vi "Lab Panel V4.86.vi"() -> ()   [LabVIEW 2013] (continued)
                            n1529 = local write "DISP LAB03-2"(w2752) -> ()
                            n1530 = local write "run lab03-2"(w2749) -> ()
                          }
                          frame #1 {
                            n1531 = TDMS Close(11:w2753) -> (0:w2754:errorcluster)  [unwired: 1 in, 1 out]
                            n1532 = local write "data file error"(w2754) -> ()
                          }
                          frame #2 {
                            n1533 = stacked-sequence {
                              tunnel: "LAB03-2" -> [w2762 w2763]
                              tunnel: w2759 -> [_ w2768]
                              tunnel: w2758 -> [_ w2767]
                              tunnel: w2757 -> [_ w2766]
                              tunnel: w2756 -> [_ w2765]
                              tunnel: w2755 -> [_ w2764]
                              frame #0 {
                                n1534 = call "sub vi - defrag tdms v1.vi"("panel id"=w2762) -> ("error out"=w2761:errorcluster)  [unwired: 10 in]
                                n1535 = local write "data file error"(w2761) -> ()
                              }
                              frame #1 {
                                n1536 = Bundle("STATUS"=w2768, "OUT SERVER ADDRESS"=w2767, "FROM ACCOUNT"=w2766, "Mail Test File To:"=w2765, "Mail Test Fail"=w2764) -> (w2770:T23)  [unwired: 1 in]
                                n1537 = call "Save data file to network drive v3.vi"("Input Cluster"=w2770, "panel id"=w2763) -> ("network file save error"=w2769:errorcluster)  [unwired: 8 in, 1 out]
                                n1538 = local write "data file error"(w2769) -> ()
                              }
                            }
                          }
                        }
                      }
                    }
                  }
                }
              }
              frame #6 {
                # "LAB04-1"
                n1539 = local read "run lab04-1"() -> (w2775:bool)
                n1540 = case shown="True" w2775 {
                  tunnel: w2774 -> [_ w2779]
                  tunnel: w2773 -> [_ w2778]
                  tunnel: w2772 -> [_ w2777]
                  tunnel: w2771 -> [_ w2776]
                  frame False {
                  }
                  frame True {
                    n1541 = local read "DISP LAB04-1"() -> (w2787:T4)
                    n1542 = Unbundle(w2787) -> ("CYCLE"=w2783:dbl, "STATUS"=w2780:string)  [unwired: 1 out]
                    n1543 = local read "TDMS LAB04-1"() -> (w2786:refnum<k34>)
                    n1544 = Not Equal?(x=w2780, y="RUN") -> (x != y?=w2782:bool)
                    n1545 = Greater?(x=w2783, y=2.0) -> (0:w2784:bool)
                    n1546 = And(x=w2784, y=w2782) -> (x .and. y?=w2781:bool)
                    n1547 = case shown="True" w2781 {
                      tunnel: w2787 -> [_ w2795]
                      tunnel: w2786 -> [_ w2794]
                      tunnel: w2780 -> [_ w2793]
                      tunnel: w2779 -> [_ w2792]
                      tunnel: w2778 -> [_ w2791]
                      tunnel: w2777 -> [_ w2790]
                      tunnel: w2776 -> [_ w2789]
                      frame False {
                      }
                      frame True {
                        n1548 = stacked-sequence {
                          tunnel: w2795 -> [w2798 _ _]
                          tunnel: w2794 -> [_ w2800 _]
                          tunnel: w2793 -> [_ _ w2806]
                          tunnel: w2792 -> [_ _ w2805]
                          tunnel: w2791 -> [_ _ w2804]
                          tunnel: w2790 -> [_ _ w2803]
                          tunnel: w2789 -> [_ _ w2802]
                          frame #0 {
                            w2796 = FALSE
                            n1549 = local write "mail control"("END") -> ()
                            n1550 = Bundle(cluster=w2798) -> (w2799:T4)  [unwired: 3 in]
                            n1551 = local write "RUN LAB04-1"(w2796) -> ()
                            n1552 = local write "O/I  LAB04-1"(w2796) -> ()
                            n1553 = local write "run lab04-1"(w2796) -> ()
                            n1554 = local write "DISP LAB04-1"(w2799) -> ()
                          }
                          frame #1 {
                            n1555 = TDMS Close(11:w2800) -> (0:w2801:errorcluster)  [unwired: 1 in, 1 out]
                            n1556 = local write "data file error"(w2801) -> ()
                          }
                          frame #2 {
                            n1557 = stacked-sequence {
                              tunnel: "LAB04-1" -> [w2809 w2810]
                              tunnel: w2806 -> [_ w2815]
                              tunnel: w2805 -> [_ w2814]
                              tunnel: w2804 -> [_ w2813]
                              tunnel: w2803 -> [_ w2812]
                              tunnel: w2802 -> [_ w2811]
                              frame #0 {
                                n1558 = call "sub vi - defrag tdms v1.vi"("panel id"=w2809) -> ("error out"=w2808:errorcluster)  [unwired: 10 in]
                                n1559 = local write "data file error"(w2808) -> ()
                              }
                              frame #1 {
                                n1560 = Bundle("STATUS"=w2815, "OUT SERVER ADDRESS"=w2814, "FROM ACCOUNT"=w2813, "Mail Test File To:"=w2812, "Mail Test Fail"=w2811) -> (w2817:T23)  [unwired: 1 in]
                                n1561 = call "Save data file to network drive v3.vi"("Input Cluster"=w2817, "panel id"=w2810) -> ("network file save error"=w2816:errorcluster)  [unwired: 8 in, 1 out]
                                n1562 = local write "data file error"(w2816) -> ()
                              }
                            }
                          }
                        }
                      }
                    }
                  }
                }
              }
              frame #7 {
                # "LAB04-2"
                n1563 = local read "run lab04-2"() -> (w2822:bool)
                n1564 = case shown="True" w2822 {
                  tunnel: w2821 -> [_ w2826]
                  tunnel: w2820 -> [_ w2825]
                  tunnel: w2819 -> [_ w2824]
                  tunnel: w2818 -> [_ w2823]
                  frame False {
                  }
                  frame True {
                    n1565 = local read "DISP LAB04-2"() -> (w2834:T4)
                    n1566 = Unbundle(w2834) -> ("CYCLE"=w2830:dbl, "STATUS"=w2827:string)  [unwired: 1 out]
                    n1567 = Not Equal?(x=w2827, y="RUN") -> (x != y?=w2829:bool)
                    n1568 = local read "TDMS LAB04-2"() -> (w2833:refnum<k34>)
                    n1569 = Greater?(x=w2830, y=2.0) -> (0:w2831:bool)
                    n1570 = And(x=w2831, y=w2829) -> (x .and. y?=w2828:bool)
                    n1571 = case shown="True" w2828 {
                      tunnel: w2834 -> [_ w2842]
                      tunnel: w2833 -> [_ w2841]
                      tunnel: w2827 -> [_ w2840]
                      tunnel: w2826 -> [_ w2839]
                      tunnel: w2825 -> [_ w2838]
                      tunnel: w2824 -> [_ w2837]
                      tunnel: w2823 -> [_ w2836]
                      frame False {
                      }
                      frame True {
                        n1572 = stacked-sequence {
                          tunnel: w2842 -> [w2845 _ _]
                          tunnel: w2841 -> [_ w2847 _]
                          tunnel: w2840 -> [_ _ w2853]
                          tunnel: w2839 -> [_ _ w2852]
                          tunnel: w2838 -> [_ _ w2851]
                          tunnel: w2837 -> [_ _ w2850]
                          tunnel: w2836 -> [_ _ w2849]
                          frame #0 {
                            w2843 = FALSE
                            n1573 = local write "mail control"("END") -> ()
                            n1574 = Bundle(cluster=w2845) -> (w2846:T4)  [unwired: 3 in]
                            n1575 = local write "O/I  LAB04-2"(w2843) -> ()
                            n1576 = local write "RUN LAB04-2"(w2843) -> ()
                            n1577 = local write "run lab04-2"(w2843) -> ()
                            n1578 = local write "DISP LAB04-2"(w2846) -> ()
                          }
                          frame #1 {
                            n1579 = TDMS Close(11:w2847) -> (0:w2848:errorcluster)  [unwired: 1 in, 1 out]
                            n1580 = local write "data file error"(w2848) -> ()
                          }
                          frame #2 {
                            n1581 = stacked-sequence {
                              tunnel: "LAB04-2" -> [w2856 w2857]
                              tunnel: w2853 -> [_ w2862]
                              tunnel: w2852 -> [_ w2861]
                              tunnel: w2851 -> [_ w2860]
                              tunnel: w2850 -> [_ w2859]
                              tunnel: w2849 -> [_ w2858]
                              frame #0 {
                                n1582 = call "sub vi - defrag tdms v1.vi"("panel id"=w2856) -> ("error out"=w2855:errorcluster)  [unwired: 10 in]
                                n1583 = local write "data file error"(w2855) -> ()
                              }
                              frame #1 {
                                n1584 = Bundle("STATUS"=w2862, "OUT SERVER ADDRESS"=w2861, "FROM ACCOUNT"=w2860, "Mail Test File To:"=w2859, "Mail Test Fail"=w2858) -> (w2864:T23)  [unwired: 1 in]
                                n1585 = call "Save data file to network drive v3.vi"("Input Cluster"=w2864, "panel id"=w2857) -> ("network file save error"=w2863:errorcluster)  [unwired: 8 in, 1 out]
                                n1586 = local write "data file error"(w2863) -> ()
                              }
                            }
                          }
                        }
                      }
                    }
                  }
                }
              }
              frame #8 {
                # "LAB05-1"
                n1587 = local read "run lab05-1"() -> (w2869:bool)
                n1588 = case shown="True" w2869 {
                  tunnel: w2868 -> [_ w2873]
                  tunnel: w2867 -> [_ w2872]
                  tunnel: w2866 -> [_ w2871]
                  tunnel: w2865 -> [_ w2870]
                  frame False {
                  }
                  frame True {
                    n1589 = local read "DISP LAB05-1"() -> (w2881:T4)
                    n1590 = Unbundle(w2881) -> ("CYCLE"=w2877:dbl, "STATUS"=w2874:string)  [unwired: 1 out]
                    n1591 = Not Equal?(x=w2874, y="RUN") -> (x != y?=w2876:bool)
                    n1592 = local read "TDMS LAB05-1"() -> (w2880:refnum<k34>)
                    n1593 = Greater?(x=w2877, y=2.0) -> (0:w2878:bool)
                    n1594 = And(x=w2878, y=w2876) -> (x .and. y?=w2875:bool)
                    n1595 = case shown="True" w2875 {
                      tunnel: w2881 -> [_ w2889]
                      tunnel: w2880 -> [_ w2888]
                      tunnel: w2874 -> [_ w2887]
                      tunnel: w2873 -> [_ w2886]
                      tunnel: w2872 -> [_ w2885]
                      tunnel: w2871 -> [_ w2884]
                      tunnel: w2870 -> [_ w2883]
                      frame False {
                      }
                      frame True {
                        n1596 = stacked-sequence {
                          tunnel: w2889 -> [w2892 _ _]
                          tunnel: w2888 -> [_ w2894 _]
                          tunnel: w2887 -> [_ _ w2900]
                          tunnel: w2886 -> [_ _ w2899]
                          tunnel: w2885 -> [_ _ w2898]
                          tunnel: w2884 -> [_ _ w2897]
                          tunnel: w2883 -> [_ _ w2896]
                          frame #0 {
                            w2890 = FALSE
                            n1597 = local write "mail control"("END") -> ()
                            n1598 = Bundle(cluster=w2892) -> (w2893:T4)  [unwired: 3 in]
                            n1599 = local write "O/I  LAB05-1"(w2890) -> ()
                            n1600 = local write "RUN LAB05-1"(w2890) -> ()
                            n1601 = local write "run lab05-1"(w2890) -> ()
                            n1602 = local write "DISP LAB05-1"(w2893) -> ()
                          }
                          frame #1 {
                            n1603 = TDMS Close(11:w2894) -> (0:w2895:errorcluster)  [unwired: 1 in, 1 out]
                            n1604 = local write "data file error"(w2895) -> ()
                          }
                          frame #2 {
                            n1605 = stacked-sequence {
                              tunnel: "LAB05-1" -> [w2903 w2909]
                              tunnel: w2900 -> [_ w2908]
                              tunnel: w2899 -> [_ w2907]
                              tunnel: w2898 -> [_ w2906]
                              tunnel: w2897 -> [_ w2905]
                              tunnel: w2896 -> [_ w2904]
                              frame #0 {
                                n1606 = call "sub vi - defrag tdms v1.vi"("panel id"=w2903) -> ("error out"=w2902:errorcluster)  [unwired: 10 in]
                                n1607 = local write "data file error"(w2902) -> ()
                              }
                              frame #1 {
                                n1608 = Bundle("STATUS"=w2908, "OUT SERVER ADDRESS"=w2907, "FROM ACCOUNT"=w2906, "Mail Test File To:"=w2905, "Mail Test Fail"=w2904) -> (w2911:T23)  [unwired: 1 in]
                                n1609 = call "Save data file to network drive v3.vi"("Input Cluster"=w2911, "panel id"=w2909) -> ("network file save error"=w2910:errorcluster)  [unwired: 8 in, 1 out]
                                n1610 = local write "data file error"(w2910) -> ()
                              }
                            }
                          }
                        }
                      }
                    }
                  }
                }
              }
              frame #9 {
                # "LAB05-2"
                n1611 = local read "run lab05-2"() -> (w2916:bool)
                n1612 = case shown="True" w2916 {
                  tunnel: w2915 -> [_ w2920]
                  tunnel: w2914 -> [_ w2919]
                  tunnel: w2913 -> [_ w2918]
                  tunnel: w2912 -> [_ w2917]
                  frame False {
                  }
                  frame True {
                    n1613 = local read "DISP LAB05-2"() -> (w2928:T4)
                    n1614 = Unbundle(w2928) -> ("CYCLE"=w2924:dbl, "STATUS"=w2921:string)  [unwired: 1 out]
                    n1615 = Not Equal?(x=w2921, y="RUN") -> (x != y?=w2923:bool)
                    n1616 = local read "TDMS LAB05-2"() -> (w2927:refnum<k34>)
                    n1617 = Greater?(x=w2924, y=2.0) -> (0:w2925:bool)
                    n1618 = And(x=w2925, y=w2923) -> (x .and. y?=w2922:bool)
                    n1619 = case shown="True" w2922 {
                      tunnel: w2928 -> [_ w2936]
                      tunnel: w2927 -> [_ w2935]
                      tunnel: w2921 -> [_ w2934]
                      tunnel: w2920 -> [_ w2933]
                      tunnel: w2919 -> [_ w2932]
                      tunnel: w2918 -> [_ w2931]
                      tunnel: w2917 -> [_ w2930]
                      frame False {
                      }
                      frame True {
                        n1620 = stacked-sequence {
                          tunnel: w2936 -> [w2939 _ _]
                          tunnel: w2935 -> [_ w2941 _]
                          tunnel: w2934 -> [_ _ w2947]
                          tunnel: w2933 -> [_ _ w2946]
                          tunnel: w2932 -> [_ _ w2945]
                          tunnel: w2931 -> [_ _ w2944]
                          tunnel: w2930 -> [_ _ w2943]
                          frame #0 {
                            w2937 = FALSE
                            n1621 = local write "mail control"("END") -> ()
                            n1622 = Bundle(cluster=w2939) -> (w2940:T4)  [unwired: 3 in]
                            n1623 = local write "RUN LAB05-2"(w2937) -> ()
                            n1624 = local write "O/I  LAB05-2"(w2937) -> ()
                            n1625 = local write "run lab05-2"(w2937) -> ()
                            n1626 = local write "DISP LAB05-2"(w2940) -> ()
                          }
                          frame #1 {
                            n1627 = TDMS Close(11:w2941) -> (0:w2942:errorcluster)  [unwired: 1 in, 1 out]
                            n1628 = local write "data file error"(w2942) -> ()
                          }
                          frame #2 {
                            n1629 = stacked-sequence {
                              tunnel: "LAB05-2" -> [w2950 w2956]
                              tunnel: w2947 -> [_ w2955]
                              tunnel: w2946 -> [_ w2954]
                              tunnel: w2945 -> [_ w2953]
                              tunnel: w2944 -> [_ w2952]
                              tunnel: w2943 -> [_ w2951]
                              frame #0 {
                                n1630 = call "sub vi - defrag tdms v1.vi"("panel id"=w2950) -> ("error out"=w2949:errorcluster)  [unwired: 10 in]
                                n1631 = local write "data file error"(w2949) -> ()
                              }
                              frame #1 {
                                n1632 = Bundle("STATUS"=w2955, "OUT SERVER ADDRESS"=w2954, "FROM ACCOUNT"=w2953, "Mail Test File To:"=w2952, "Mail Test Fail"=w2951) -> (w2958:T23)  [unwired: 1 in]
                                n1633 = call "Save data file to network drive v3.vi"("Input Cluster"=w2958, "panel id"=w2956) -> ("network file save error"=w2957:errorcluster)  [unwired: 8 in, 1 out]
                                n1634 = local write "data file error"(w2957) -> ()
                              }
                            }
                          }
                        }
                      }
                    }
                  }
                }
              }
            }
            n1635 = local read "Network Directory"() -> (w2472:path)
            n1636 = global write "Global 1.vi" "Network Drive"(w2472) -> ()
          }
          frame #7 {
            # "disable functions"
            n1637 = stacked-sequence {
              tunnel: w2968 -> [w2982 _ w3039]
              tunnel: w2967 -> [w2977 _ w3038]
              tunnel: w2966 -> [w2976 _ w3037]
              tunnel: w2965 -> [w2974 _ w3036]
              tunnel: w2964 -> [w2975 _ w3035]
              tunnel: w2963 -> [_ w2999 w3034]
              tunnel: w2962 -> [_ w3000 w3033]
              tunnel: w2961 -> [_ w3001 w3032]
              tunnel: w2960 -> [_ w3002 w3031]
              tunnel: w2959 -> [_ w3003 w3030]
              frame #0 {
                n1638 = Select(t=2, s=w2974, f=0) -> (s? t:f=w2970:i32)
                n1639 = Select(t=2, s=w2976, f=0) -> (s? t:f=w2971:i32)
                n1640 = Select(t=2, s=w2975, f=0) -> (s? t:f=w2969:i32)
                n1641 = Select(t=2, s=w2982, f=0) -> (s? t:f=w2973:i32)
                n1642 = Select(t=2, s=w2977, f=0) -> (s? t:f=w2972:i32)
                n1643 = property on="SELECT LAB02-2" class="RadioBtnsControl (strict)"("DisabledEnum"=w2970) -> ()  [unwired: 2 in, 2 out]
                n1644 = property on="SELECT LAB02-1" class="RadioBtnsControl (strict)"("DisabledEnum"=w2971) -> ()  [unwired: 2 in, 2 out]
                n1645 = property on="SELECT LAB03-1" class="RadioBtnsControl (strict)"("DisabledEnum"=w2969) -> ()  [unwired: 2 in, 2 out]
                n1646 = property on="SELECT LAB01-1" class="RadioBtnsControl (strict)"("DisabledEnum"=w2973) -> ()  [unwired: 2 in, 2 out]
                n1647 = property on="SELECT LAB01-2" class="RadioBtnsControl (strict)"("DisabledEnum"=w2972) -> ()  [unwired: 2 in, 2 out]
                n1648 = Not(x=w2982) -> (.not. x?=w2983:bool)
                n1649 = property on="RESULT LAB01-1" class="Bool (strict)"("Visible"=w2983) -> ()  [unwired: 2 in, 2 out]
                n1650 = Not(x=w2977) -> (.not. x?=w2981:bool)
                n1651 = Not(x=w2976) -> (.not. x?=w2980:bool)
                n1652 = Not(x=w2974) -> (.not. x?=w2979:bool)
                n1653 = property on="RESULT LAB01-2" class="Bool (strict)"("Visible"=w2981) -> ()  [unwired: 2 in, 2 out]
                n1654 = Not(x=w2975) -> (.not. x?=w2978:bool)
                n1655 = property on="RESULT LAB02-1" class="Bool (strict)"("Visible"=w2980) -> ()  [unwired: 2 in, 2 out]
                n1656 = property on="RESULT LAB02-2" class="Bool (strict)"("Visible"=w2979) -> ()  [unwired: 2 in, 2 out]
                n1657 = property on="RESULT LAB03-1" class="Bool (strict)"("Visible"=w2978) -> ()  [unwired: 2 in, 2 out]
                n1658 = property on="SET LAB01-1" class="Clust (strict)"("DisabledEnum"=w2973) -> ()  [unwired: 2 in, 2 out]
                n1659 = property on="SET LAB01-2" class="Clust (strict)"("DisabledEnum"=w2972) -> ()  [unwired: 2 in, 2 out]
                n1660 = property on="SET LAB02-1" class="Clust (strict)"("DisabledEnum"=w2971) -> ()  [unwired: 2 in, 2 out]
                n1661 = property on="SET LAB02-2" class="Clust (strict)"("DisabledEnum"=w2970) -> ()  [unwired: 2 in, 2 out]
                n1662 = property on="SET LAB03-1" class="Clust (strict)"("DisabledEnum"=w2969) -> ()  [unwired: 2 in, 2 out]
                n1663 = property on="O/I  LAB01-1" class="Bool (strict)"("DisabledEnum"=w2973) -> ()  [unwired: 2 in, 2 out]
                n1664 = property on="O/I  LAB01-2" class="Bool (strict)"("DisabledEnum"=w2972) -> ()  [unwired: 2 in, 2 out]
                n1665 = property on="O/I  LAB02-1" class="Bool (strict)"("DisabledEnum"=w2971) -> ()  [unwired: 2 in, 2 out]
                n1666 = property on="O/I  LAB02-2" class="Bool (strict)"("DisabledEnum"=w2970) -> ()  [unwired: 2 in, 2 out]
                n1667 = property on="O/I  LAB03-1" class="Bool (strict)"("DisabledEnum"=w2969) -> ()  [unwired: 2 in, 2 out]
              }
              frame #1 {
                n1668 = Select(t=2, s=w3003, f=0) -> (s? t:f=w2994:i32)
                n1669 = Select(t=2, s=w3002, f=0) -> (s? t:f=w2995:i32)
                n1670 = Select(t=2, s=w2999, f=0) -> (s? t:f=w2998:i32)
                n1671 = Select(t=2, s=w3000, f=0) -> (s? t:f=w2997:i32)
                n1672 = Select(t=2, s=w3001, f=0) -> (s? t:f=w2996:i32)
                n1673 = property on="SELECT LAB05-2" class="RadioBtnsControl (strict)"("DisabledEnum"=w2994) -> ()  [unwired: 2 in, 2 out]
                n1674 = property on="SELECT LAB05-1" class="RadioBtnsControl (strict)"("DisabledEnum"=w2995) -> ()  [unwired: 2 in, 2 out]
                n1675 = property on="SELECT LAB03-2" class="RadioBtnsControl (strict)"("DisabledEnum"=w2998) -> ()  [unwired: 2 in, 2 out]
                n1676 = property on="SELECT LAB04-1" class="RadioBtnsControl (strict)"("DisabledEnum"=w2997) -> ()  [unwired: 2 in, 2 out]
                n1677 = property on="SELECT LAB04-2" class="RadioBtnsControl (strict)"("DisabledEnum"=w2996) -> ()  [unwired: 2 in, 2 out]
                n1678 = property on="SET LAB05-2" class="Clust (strict)"("DisabledEnum"=w2994) -> ()  [unwired: 2 in, 2 out]
                n1679 = property on="SET LAB05-1" class="Clust (strict)"("DisabledEnum"=w2995) -> ()  [unwired: 2 in, 2 out]
                n1680 = property on="SET LAB03-2" class="Clust (strict)"("DisabledEnum"=w2998) -> ()  [unwired: 2 in, 2 out]
                n1681 = property on="SET LAB04-1" class="Clust (strict)"("DisabledEnum"=w2997) -> ()  [unwired: 2 in, 2 out]
                n1682 = property on="SET LAB04-2" class="Clust (strict)"("DisabledEnum"=w2996) -> ()  [unwired: 2 in, 2 out]
                n1683 = property on="O/I  LAB05-2" class="Bool (strict)"("DisabledEnum"=w2994) -> ()  [unwired: 2 in, 2 out]
                n1684 = property on="O/I  LAB05-1" class="Bool (strict)"("DisabledEnum"=w2995) -> ()  [unwired: 2 in, 2 out]
                n1685 = property on="O/I  LAB04-1" class="Bool (strict)"("DisabledEnum"=w2997) -> ()  [unwired: 2 in, 2 out]
                n1686 = property on="O/I  LAB04-2" class="Bool (strict)"("DisabledEnum"=w2996) -> ()  [unwired: 2 in, 2 out]
                n1687 = property on="O/I  LAB03-2" class="Bool (strict)"("DisabledEnum"=w2998) -> ()  [unwired: 2 in, 2 out]
                n1688 = Not(x=w3003) -> (.not. x?=w3004:bool)
                n1689 = Not(x=w3002) -> (.not. x?=w3005:bool)
                n1690 = Not(x=w3001) -> (.not. x?=w3006:bool)
                n1691 = property on="RESULT LAB05-2" class="Bool (strict)"("Visible"=w3004) -> ()  [unwired: 2 in, 2 out]
                n1692 = property on="RESULT LAB05-1" class="Bool (strict)"("Visible"=w3005) -> ()  [unwired: 2 in, 2 out]
                n1693 = Not(x=w3000) -> (.not. x?=w3007:bool)
                n1694 = property on="RESULT LAB04-2" class="Bool (strict)"("Visible"=w3006) -> ()  [unwired: 2 in, 2 out]
                n1695 = Not(x=w2999) -> (.not. x?=w3008:bool)
                n1696 = property on="RESULT LAB04-1" class="Bool (strict)"("Visible"=w3007) -> ()  [unwired: 2 in, 2 out]
                n1697 = property on="RESULT LAB03-2" class="Bool (strict)"("Visible"=w3008) -> ()  [unwired: 2 in, 2 out]
              }
              frame #2 {
                # "disable calibrate if any test running"
                n1698 = Or(x=w3031, y=w3030) -> (x .or. y?=w3024:bool)
                n1699 = Or(x=w3033, y=w3032) -> (x .or. y?=w3026:bool)
                n1700 = Or(x=w3037, y=w3036) -> (x .or. y?=w3028:bool)
                n1701 = Or(x=w3035, y=w3034) -> (x .or. y?=w3027:bool)
                n1702 = Or(x=w3039, y=w3038) -> (x .or. y?=w3029:bool)
                n1703 = Or(x=w3027, y=w3026) -> (x .or. y?=w3025:bool)
                n1704 = Or(x=w3029, y=w3028) -> (x .or. y?=w3023:bool)
                n1705 = Or(x=w3025, y=w3024) -> (x .or. y?=w3022:bool)
                n1706 = Or(x=w3023, y=w3022) -> (x .or. y?=w3021:bool)
                n1707 = case shown="False" w3021 {
                  tunnel: [0 2] -> w3020
                  frame False {
                  }
                  frame True {
                  }
                }
                n1708 = property on="JIG TEST" class="Clust (strict)"("DisabledEnum"=w3020) -> ()  [unwired: 2 in, 2 out]
                n1709 = property on="Network Directory" class="Path"("DisabledEnum"=w3020) -> ()  [unwired: 2 in, 2 out]
                n1710 = property on="MAIL SETTINGS" class="Clust (strict)"("DisabledEnum"=w3020) -> ()  [unwired: 2 in, 2 out]
                n1711 = property on="SET (cal)" class="Bool (strict)"("DisabledEnum"=w3020) -> ()  [unwired: 2 in, 2 out]
                n1712 = property on="ADMIN" class="Bool (strict)"("DisabledEnum"=0) -> ()  [unwired: 2 in, 2 out]
              }
            }
          }
          frame #8 {
            # "drive jigs"
            n1713 = stacked-sequence {
              frame #0 {
                # "jig on"
                n1714 = local read "jig cycle"() -> (w3047:dbl)
                n1715 = property on="JIG TEST" class="Clust (strict)"() -> ("DisabledEnum"=w3044:T14)  [unwired: 2 in, 2 out]
                n1716 = Equal?(x=w3044, y=2) -> (x = y?=w3043:bool)
                n1717 = Equal?(x=w3047, y=0) -> (x = y?=w3045:bool)
                n1718 = And(x=w3045, y=w3043) -> (x .and. y?=w3042:bool)
                n1719 = case shown="True" w3042 {
                  frame False {
                  }
                  frame True {
                    n1720 = local read "run lab01-1"() -> (w3058:bool)
                    n1721 = local read "run lab01-2"() -> (w3057:bool)
                    n1722 = local read "run lab02-1"() -> (w3056:bool)
                    n1723 = local read "run lab02-2"() -> (w3055:bool)
                    n1724 = local read "run lab03-1"() -> (w3054:bool)
                    n1725 = local read "run lab03-2"() -> (w3053:bool)
                    n1726 = local read "run lab04-1"() -> (w3052:bool)
                    n1727 = local read "run lab04-2"() -> (w3051:bool)
                    n1728 = local read "run lab05-1"() -> (w3050:bool)
                    n1729 = local read "run lab05-2"() -> (w3049:bool)
                    n1730 = local write "JIG LAB03-2"(w3053) -> ()
                    n1731 = local write "JIG LAB01-1"(w3058) -> ()
                    n1732 = local write "JIG LAB01-2"(w3057) -> ()
                    n1733 = local write "JIG LAB02-1"(w3056) -> ()
                    n1734 = local write "JIG LAB02-2"(w3055) -> ()
                    n1735 = local write "JIG LAB03-1"(w3054) -> ()
                    n1736 = local write "JIG LAB04-1"(w3052) -> ()
                    n1737 = local write "JIG LAB04-2"(w3051) -> ()
                    n1738 = local write "JIG LAB05-1"(w3050) -> ()
                    n1739 = local write "JIG LAB05-2"(w3049) -> ()
                  }
                }
              }
              frame #1 {
                # "jig off"
                n1740 = local read "jig cycle"() -> (w3065:dbl)
                n1741 = local read "on loops"() -> (w3064:dbl)
                n1742 = property on="JIG TEST" class="Clust (strict)"() -> ("DisabledEnum"=w3063:T14)  [unwired: 2 in, 2 out]
                n1743 = Equal?(x=w3063, y=2) -> (x = y?=w3061:bool)
                n1744 = Equal?(x=w3065, y=w3064) -> (x = y?=w3060:bool)
                n1745 = And(x=w3060, y=w3061) -> (x .and. y?=w3059:bool)
                n1746 = case shown="True" w3059 {
                  frame False {
                  }
                  frame True {
                    w3116 = FALSE
                    w3117 = TRUE
                    w3115 = 2
                    n1747 = local read "SELECT LAB05-2"() -> (w3106:T3)
                    n1748 = local read "SELECT LAB04-2"() -> (w3108:T3)
                    n1749 = local read "SELECT LAB04-1"() -> (w3109:T3)
                    n1750 = local read "SELECT LAB05-1"() -> (w3107:T3)
                    n1751 = local read "SELECT LAB03-2"() -> (w3110:T3)
                    n1752 = local read "SELECT LAB02-1"() -> (w3113:T3)
                    n1753 = local read "SELECT LAB03-1"() -> (w3111:T3)
                    n1754 = local read "SELECT LAB02-2"() -> (w3112:T3)
                    n1755 = local read "SELECT LAB01-2"() -> (w3114:T3)
                    n1756 = local read "run lab05-1"() -> (w3076:bool)
                    n1757 = local read "run lab05-2"() -> (w3075:bool)
                    n1758 = local read "SELECT LAB01-1"() -> (w3118:T3)
                    n1759 = local read "run lab04-2"() -> (w3077:bool)
                    n1760 = local read "run lab04-1"() -> (w3078:bool)
                    n1761 = local read "run lab01-1"() -> (w3094:bool)
                    n1762 = local read "run lab01-2"() -> (w3083:bool)
                    n1763 = local read "run lab03-2"() -> (w3079:bool)
                    n1764 = local read "run lab03-1"() -> (w3080:bool)
                    n1765 = local read "run lab02-1"() -> (w3082:bool)
                    n1766 = local read "run lab02-2"() -> (w3081:bool)
                    n1767 = Equal?(x=w3115, y=w3111) -> (x = y?=w3089:bool)
                    n1768 = Equal?(x=w3115, y=w3110) -> (x = y?=w3088:bool)
                    n1769 = Equal?(x=w3115, y=w3109) -> (x = y?=w3087:bool)
                    n1770 = Equal?(x=w3115, y=w3108) -> (x = y?=w3086:bool)
                    n1771 = Equal?(x=w3115, y=w3107) -> (x = y?=w3085:bool)
                    n1772 = Equal?(x=w3115, y=w3106) -> (x = y?=w3084:bool)
                    n1773 = Equal?(x=w3115, y=w3118) -> (x = y?=w3095:bool)
                    n1774 = Equal?(x=w3115, y=w3113) -> (x = y?=w3091:bool)
                    n1775 = Equal?(x=w3115, y=w3112) -> (x = y?=w3090:bool)
                    n1776 = Equal?(x=w3115, y=w3114) -> (x = y?=w3092:bool)
                    n1777 = And(x=w3086, y=w3077) -> (x .and. y?=w3068:bool)
                    n1778 = And(x=w3089, y=w3080) -> (x .and. y?=w3071:bool)
                    n1779 = And(x=w3087, y=w3078) -> (x .and. y?=w3069:bool)
                    n1780 = And(x=w3084, y=w3075) -> (x .and. y?=w3066:bool)
                    n1781 = And(x=w3090, y=w3081) -> (x .and. y?=w3072:bool)
                    n1782 = And(x=w3088, y=w3079) -> (x .and. y?=w3070:bool)
                    n1783 = And(x=w3085, y=w3076) -> (x .and. y?=w3067:bool)
                    n1784 = And(x=w3092, y=w3083) -> (x .and. y?=w3074:bool)
                    n1785 = And(x=w3095, y=w3094) -> (x .and. y?=w3093:bool)
                    n1786 = And(x=w3091, y=w3082) -> (x .and. y?=w3073:bool)
                    n1787 = Select(t=w3117, s=w3093, f=w3116) -> (s? t:f=w3096:bool)
                    n1788 = Select(t=w3117, s=w3074, f=w3116) -> (s? t:f=w3097:bool)
                    n1789 = Select(t=w3117, s=w3073, f=w3116) -> (s? t:f=w3098:bool)
                    n1790 = Select(t=w3117, s=w3072, f=w3116) -> (s? t:f=w3099:bool)
                    n1791 = Select(t=w3117, s=w3071, f=w3116) -> (s? t:f=w3100:bool)
                    n1792 = Select(t=w3117, s=w3070, f=w3116) -> (s? t:f=w3101:bool)
                    n1793 = Select(t=w3117, s=w3069, f=w3116) -> (s? t:f=w3102:bool)
                    n1794 = Select(t=w3117, s=w3068, f=w3116) -> (s? t:f=w3103:bool)
                    n1795 = Select(t=w3117, s=w3067, f=w3116) -> (s? t:f=w3104:bool)
                    n1796 = Select(t=w3117, s=w3066, f=w3116) -> (s? t:f=w3105:bool)
                    n1797 = local write "JIG LAB03-2"(w3101) -> ()
                    n1798 = local write "JIG LAB02-1"(w3098) -> ()
                    n1799 = local write "JIG LAB02-2"(w3099) -> ()
                    n1800 = local write "JIG LAB01-2"(w3097) -> ()
                    n1801 = local write "JIG LAB03-1"(w3100) -> ()
                    n1802 = local write "JIG LAB01-1"(w3096) -> ()
                    n1803 = local write "JIG LAB05-2"(w3105) -> ()
                    n1804 = local write "JIG LAB04-1"(w3102) -> ()
                    n1805 = local write "JIG LAB05-1"(w3104) -> ()
                    n1806 = local write "JIG LAB04-2"(w3103) -> ()
                  }
                }
              }
            }
          }
          frame #9 {
            # "enable  jig test output if no test busy"
            n1807 = property on="JIG TEST" class="Clust (strict)"() -> ("DisabledEnum"=w3121:T14)  [unwired: 2 in, 2 out]
            n1808 = Equal?(x=w3121, y=0) -> (x = y?=w3119:bool)
            n1809 = case shown="True" w3119 {
              frame False {
              }
              frame True {
                n1810 = local read "JIG TEST"() -> (w3132:T9)
                n1811 = Unbundle(w3132) -> ("LAB01-1"=w3131:bool, "LAB01-2"=w3130:bool, "LAB02-1"=w3129:bool, "LAB02-2"=w3128:bool, "LAB03-1"=w3127:bool, "LAB03-2"=w3126:bool, "LAB04-1"=w3125:bool, "LAB04-2"=w3124:bool, "LAB05-1"=w3123:bool, "LAB05-2"=w3122:bool)
                n1812 = local write "JIG LAB05-1"(w3123) -> ()
                n1813 = local write "JIG LAB05-2"(w3122) -> ()
                n1814 = local write "JIG LAB04-1"(w3125) -> ()
                n1815 = local write "JIG LAB04-2"(w3124) -> ()
                n1816 = local write "JIG LAB03-2"(w3126) -> ()
                n1817 = local write "JIG LAB01-1"(w3131) -> ()
                n1818 = local write "JIG LAB02-1"(w3129) -> ()
                n1819 = local write "JIG LAB03-1"(w3127) -> ()
                n1820 = local write "JIG LAB01-2"(w3130) -> ()
                n1821 = local write "JIG LAB02-2"(w3128) -> ()
              }
            }
          }
          frame #10 {
            # "drive digital output"
            n1822 = local read "O/I  LAB05-2"() -> (w3139:bool)
            n1823 = local read "O/I  LAB05-1"() -> (w3141:bool)
            n1824 = local read "JIG LAB05-2"() -> (w3138:bool)
            n1825 = local read "O/I  LAB04-2"() -> (w3143:bool)
            n1826 = local read "JIG LAB05-1"() -> (w3140:bool)
            n1827 = local read "JIG LAB04-2"() -> (w3142:bool)
            n1828 = local read "O/I  LAB03-1"() -> (w3148:bool)
            n1829 = local read "O/I  LAB04-1"() -> (w3144:bool)
            n1830 = local read "O/I  LAB02-1"() -> (w3152:bool)
            n1831 = local read "O/I  LAB02-2"() -> (w3150:bool)
            n1832 = local read "O/I  LAB03-2"() -> (w3146:bool)
            n1833 = local read "JIG LAB04-1"() -> (w3137:bool)
            n1834 = local read "JIG LAB03-2"() -> (w3145:bool)
            n1835 = local read "O/I  LAB01-2"() -> (w3154:bool)
            n1836 = local read "JIG LAB02-1"() -> (w3151:bool)
            n1837 = local read "JIG LAB02-2"() -> (w3149:bool)
            n1838 = local read "JIG LAB03-1"() -> (w3147:bool)
            n1839 = local read "O/I  LAB01-1"() -> (w3156:bool)
            n1840 = local read "JIG LAB01-2"() -> (w3153:bool)
            n1841 = local read "JIG LAB01-1"() -> (w3155:bool)
            n1842 = Build Array(w3143, w3142, w3141, w3140, w3139, w3138) -> (w3134:bool[])
            n1843 = Build Array(w3149, w3148, w3147, w3146, w3145, w3144, w3137) -> (w3135:bool[])
            n1844 = Build Array(w3156, w3155, w3154, w3153, w3152, w3151, w3150) -> (w3136:bool[])
            n1845 = local read "simulate"() -> (w3133:bool)
            n1846 = case shown="False" w3133 {
              tunnel: w3136 -> [w3159 _]
              tunnel: w3135 -> [w3158 _]
              tunnel: w3134 -> [w3157 _]
              frame False {
                n1847 = call "sub vi - Drive Relays All v6.vi"("Array #2"=w3157, "Array #1"=w3158, "Array #0"=w3159) -> ()  [unwired: 8 in, 1 out]
              }
              frame True {
              }
            }
          }
          frame #11 {
            # "get analog values"
            n1848 = local read "on loops"() -> (w3166:dbl)
            n1849 = local read "jig cycle"() -> (w3163:dbl)
            n1850 = Add(x=w3166, y=1) -> (x+y=w3164:dbl)
            n1851 = Equal?(x=w3163, y=1) -> (x = y?=w3160:bool)
            n1852 = Equal?(x=w3163, y=w3164) -> (x = y?=w3162:bool)
            n1853 = Or(x=w3160, y=w3162) -> (x .or. y?=w3161:bool)
            n1854 = global write "Global display 3.vi" "cycle O/F"(w3160) -> ()
            n1855 = case shown="True" w3161 {
              frame False {
              }
              frame True {
                n1856 = local read "simulate"() -> (w3170:bool)
                n1857 = case shown="False" w3170 {
                  tunnel: [w3179 errorcluster[] [] ("array ERROR")] -> w3178
                  tunnel: [w3186 0.3 ("Analog loop time")] -> w3177
                  tunnel: [w3185 dynamicdata[] [] ("array GRAPH")] -> w3176
                  tunnel: [w3184 w3188] -> w3175
                  tunnel: [w3183 w3188] -> w3174
                  tunnel: [w3182 w3188] -> w3173
                  tunnel: [w3181 w3188] -> w3172
                  tunnel: [w3180 w3188] -> w3171
                  frame False {
                    n1858 = call "sub vi - Read Analog All v8.11.vi"() -> ("Analog loop time"=w3186:dbl, "array GRAPH"=w3185:dynamicdata[], "LAB01"=w3184:T24, "LAB02"=w3183:T25, "LAB03"=w3182:T26, "LAB04"=w3181:T27, "array ERROR"=w3179:errorcluster[], "LAB05"=w3180:T28)  [unwired: 8 in]
                  }
                  frame True {
                    w3188 = T28 {"LAB05-1 (A)"=10.0, "LAB05-1 (V)"=220.0, "LAB05-1 (PF)"=0.5, "LAB05-2 (A)"=15.0, "LAB05-2 (V)"=225.0, "LAB05-2 (PF)"=0.6} ("LAB05")
                  }
                }
                n1859 = local read "simulate"() -> (w3169:bool)
                n1860 = stacked-sequence {
                  tunnel: w3178 -> [w3195 _ _ _ _ _]
                  tunnel: w3177 -> [w3194 _ _ _ _ _]
                  tunnel: w3176 -> [w3191 _ _ _ _ _]
                  tunnel: w3175 -> [_ w3242 _ _ _ _]
                  tunnel: w3174 -> [_ _ w3249 _ _ _]
                  tunnel: w3173 -> [_ _ _ w3278 _ _]
                  tunnel: w3172 -> [_ _ _ _ w3305 _]
                  tunnel: w3171 -> [_ _ _ _ _ w3334]
                  tunnel: w3169 -> [_ w3220 w3248 w3276 w3304 w3332]
                  tunnel: T12 {"1  (A) cal"=1.0, "1 (V) cal"=1.0, "1 (PF) cal"=1.0, "1 (TL) cal"=1.0, "1 (TN) cal"=1.0, "2 (A) cal"=1.0, "2 (V) cal"=1.0, "2 (PF) cal"=1.0, "2 (TL) cal"=1.0, "2 (TN) cal"=1.0} ("CAL LAB01") -> [_ w3219 w3247 w3275 w3303 w3331]
                  frame #0 {
                    n1861 = local write "AI"(TRUE) -> ()
                    n1862 = global write "Global 1.vi" "RATE(Hz)"("RATE (Hz)") -> ()
                    n1863 = global write "Global 1.vi" "SAMPLES"("SAMPLES") -> ()
                    n1864 = Index Array(array=w3191, index=6) -> (element=→"LAB04-1 (GRAPH)":dynamicdata)
                    n1865 = Index Array(array=w3191, index=7) -> (element=→"LAB04-2 (GRAPH)":dynamicdata)
                    n1866 = Index Array(array=w3191, index=9) -> (element=→"LAB05-2 (GRAPH)":dynamicdata)
                    n1867 = Index Array(array=w3191, index=8) -> (element=→"LAB05-1 (GRAPH)":dynamicdata)
                    n1868 = Index Array(array=w3191, index=5) -> (element=→"LAB03-2 (GRAPH)":dynamicdata)
                    n1869 = Index Array(array=w3191, index=0) -> (element=→"LAB01-1 (GRAPH)":dynamicdata)
                    n1870 = Index Array(array=w3191, index=1) -> (element=→"LAB01-2 (GRAPH)":dynamicdata)
                    n1871 = Index Array(array=w3191, index=2) -> (element=→"LAB02-1 (GRAPH)":dynamicdata)
                    n1872 = Index Array(array=w3191, index=3) -> (element=→"LAB02-2 (GRAPH)":dynamicdata)
                    n1873 = Index Array(array=w3191, index=4) -> (element=→"LAB03-1 (GRAPH)":dynamicdata)
                    "AI loop time" <- w3194
                    "Analog Error Array" <- w3195
                  }
                  frame #1 {
                    n1874 = Unbundle By Name(w3242) -> ("LAB05-1 (A)"=w3240:dbl, "LAB05-1 (V)"=w3239:dbl, "LAB05-1 (PF)"=w3238:dbl, "LAB05-2 (A)"=w3237:dbl, "LAB05-2 (V)"=w3236:dbl, "LAB05-2 (PF)"=w3235:dbl)
                    n1875 = case shown="False" w3220 {
                      tunnel: [w3243 w3244] -> w3241
                      tunnel: w3219 -> [_ w3244]
                      frame False {
                        n1876 = local read "CAL LAB01"() -> (w3243:T12)
                      }
                      frame True {
                      }
                    }
                    n1877 = Unbundle By Name(w3241) -> ("1  (A) cal"=w3234:dbl, "1 (V) cal"=w3233:dbl, "1 (PF) cal"=w3232:dbl, "2 (A) cal"=w3231:dbl, "2 (V) cal"=w3230:dbl, "2 (PF) cal"=w3229:dbl)  [unwired: 4 out]
                    n1878 = Multiply(x=w3240, y=w3234) -> (x*y=w3227:dbl)
                    n1879 = Multiply(x=w3239, y=w3233) -> (x*y=w3226:dbl)
                    n1880 = Multiply(x=w3238, y=w3232) -> (x*y=w3225:dbl)
                    n1881 = Multiply(x=w3237, y=w3231) -> (x*y=w3223:dbl)
                    n1882 = Multiply(x=w3236, y=w3230) -> (x*y=w3222:dbl)
                    n1883 = Multiply(x=w3235, y=w3229) -> (x*y=w3221:dbl)
                    n1884 = local read "SIG LAB01-1"() -> (w3228:T2)
                    n1885 = local read "SIG LAB01-2"() -> (w3224:T2)
                    n1886 = Bundle By Name(cluster=w3228, "AMPS"=w3227, "VOLTS"=w3226, "PF"=w3225) -> (w3218:T2)
                    n1887 = Bundle By Name(cluster=w3224, "AMPS"=w3223, "VOLTS"=w3222, "PF"=w3221) -> (w3217:T2)
                    n1888 = global write "Global display 1.vi" "SIG LAB01-2"(w3217) -> ()
                    n1889 = global write "Global display 1.vi" "SIG LAB01-1"(w3218) -> ()
                    n1890 = local write "SIG LAB01-2"(w3217) -> ()
                    n1891 = local write "SIG LAB01-1"(w3218) -> ()
                  }
                  frame #2 {
                    n1892 = Unbundle By Name(w3249) -> ("LAB05-1 (A)"=w3269:dbl, "LAB05-1 (V)"=w3268:dbl, "LAB05-1 (PF)"=w3267:dbl, "LAB05-2 (A)"=w3266:dbl, "LAB05-2 (V)"=w3265:dbl, "LAB05-2 (PF)"=w3264:dbl)
                    n1893 = case shown="True" w3248 {
                      tunnel: [w3271 w3272] -> w3270
                      tunnel: w3247 -> [_ w3272]
                      frame False {
                        n1894 = local read "CAL LAB02"() -> (w3271:T13)
                      }
                      frame True {
                      }
                    }
                    n1895 = Unbundle By Name(w3270) -> ("1  (A) cal"=w3263:dbl, "1 (V) cal"=w3262:dbl, "1 (PF) cal"=w3261:dbl, "2 (A) cal"=w3260:dbl, "2 (V) cal"=w3259:dbl, "2 (PF) cal"=w3258:dbl)  [unwired: 4 out]
                    n1896 = Multiply(x=w3269, y=w3263) -> (x*y=w3256:dbl)
                    n1897 = Multiply(x=w3268, y=w3262) -> (x*y=w3255:dbl)
                    n1898 = Multiply(x=w3267, y=w3261) -> (x*y=w3254:dbl)
                    n1899 = Multiply(x=w3266, y=w3260) -> (x*y=w3252:dbl)
                    n1900 = Multiply(x=w3265, y=w3259) -> (x*y=w3251:dbl)
                    n1901 = Multiply(x=w3264, y=w3258) -> (x*y=w3250:dbl)
                    n1902 = local read "SIG LAB02-1"() -> (w3257:T2)
                    n1903 = local read "SIG LAB02-2"() -> (w3253:T2)
                    n1904 = Bundle By Name(cluster=w3257, "AMPS"=w3256, "VOLTS"=w3255, "PF"=w3254) -> (w3246:T2)
                    n1905 = Bundle By Name(cluster=w3253, "AMPS"=w3252, "VOLTS"=w3251, "PF"=w3250) -> (w3245:T2)
                    n1906 = global write "Global display 1.vi" "SIG LAB02-1"(w3246) -> ()
                    n1907 = local write "SIG LAB02-2"(w3245) -> ()
                    n1908 = global write "Global display 1.vi" "SIG LAB02-2"(w3245) -> ()
                    n1909 = local write "SIG LAB02-1"(w3246) -> ()
                  }
                  frame #3 {
                    n1910 = Unbundle By Name(w3278) -> ("LAB05-1 (A)"=w3297:dbl, "LAB05-1 (V)"=w3296:dbl, "LAB05-1 (PF)"=w3295:dbl, "LAB05-2 (A)"=w3294:dbl, "LAB05-2 (V)"=w3293:dbl, "LAB05-2 (PF)"=w3292:dbl)
                    n1911 = case shown="True" w3276 {
                      tunnel: [w3299 w3300] -> w3298
                      tunnel: w3275 -> [_ w3300]
                      frame False {
                        n1912 = local read "CAL LAB03"() -> (w3299:T12)
                      }
                      frame True {
                      }
                    }
                    n1913 = Unbundle By Name(w3298) -> ("1  (A) cal"=w3291:dbl, "1 (V) cal"=w3290:dbl, "1 (PF) cal"=w3289:dbl, "2 (A) cal"=w3288:dbl, "2 (V) cal"=w3287:dbl, "2 (PF) cal"=w3286:dbl)  [unwired: 4 out]
                    n1914 = Multiply(x=w3297, y=w3291) -> (x*y=w3284:dbl)
                    n1915 = Multiply(x=w3296, y=w3290) -> (x*y=w3277:dbl)
                    n1916 = Multiply(x=w3295, y=w3289) -> (x*y=w3283:dbl)
                    n1917 = Multiply(x=w3294, y=w3288) -> (x*y=w3281:dbl)
                    n1918 = Multiply(x=w3293, y=w3287) -> (x*y=w3280:dbl)
                    n1919 = Multiply(x=w3292, y=w3286) -> (x*y=w3279:dbl)
                    n1920 = local read "SIG LAB03-1"() -> (w3285:T2)
                    n1921 = local read "SIG LAB03-2"() -> (w3282:T2)
                    n1922 = Bundle By Name(cluster=w3285, "AMPS"=w3284, "VOLTS"=w3277, "PF"=w3283) -> (w3274:T2)
                    n1923 = Bundle By Name(cluster=w3282, "AMPS"=w3281, "VOLTS"=w3280, "PF"=w3279) -> (w3273:T2)
                    n1924 = global write "Global display 1.vi" "SIG LAB03-1"(w3274) -> ()
                    n1925 = global write "Global display 1.vi" "SIG LAB03-2"(w3273) -> ()
                    n1926 = local write "SIG LAB03-2"(w3273) -> ()
                    n1927 = local write "SIG LAB03-1"(w3274) -> ()
                  }
                  frame #4 {
                    n1928 = Unbundle By Name(w3305) -> ("LAB05-1 (A)"=w3325:dbl, "LAB05-1 (V)"=w3324:dbl, "LAB05-1 (PF)"=w3323:dbl, "LAB05-2 (A)"=w3322:dbl, "LAB05-2 (V)"=w3321:dbl, "LAB05-2 (PF)"=w3320:dbl)
                    n1929 = case shown="False" w3304 {
                      tunnel: [w3327 w3328] -> w3326
                      tunnel: w3303 -> [_ w3328]
                      frame False {
                        n1930 = local read "CAL LAB04"() -> (w3327:T12)
                      }
